vi "widget.vi"(8 "Error In":errorcluster, 10 "index":i32, 11 "QStackedWidget In":refnum<class "QStackedWidget.lvclass">) -> (0 "Error Out":errorcluster, 2 "Value":refnum<class "QWidget.lvclass">, 3 "QStackedWidget Out":refnum<class "QStackedWidget.lvclass">)   [LabVIEW 2014, in "QStackedWidget.lvclass"]
doc: "LabVIEW-specific documentation is not yet available. See <b>https://doc.qt.io/qt-5/qstackedwidget.html#widget</b>"
uses:
  QStackedWidget.lvclass
  QWidget/QWidget.lvclass
  LQ Core/LQIdentity/LQIdentity.lvclass/LQIdentity.ctl
  LQ Core/LQ Core.lvlib
  LQ Core/LQIdentity/LQIdentity.lvclass
  LQ Core/LQCoreEngine/LQCoreEngine.lvclass
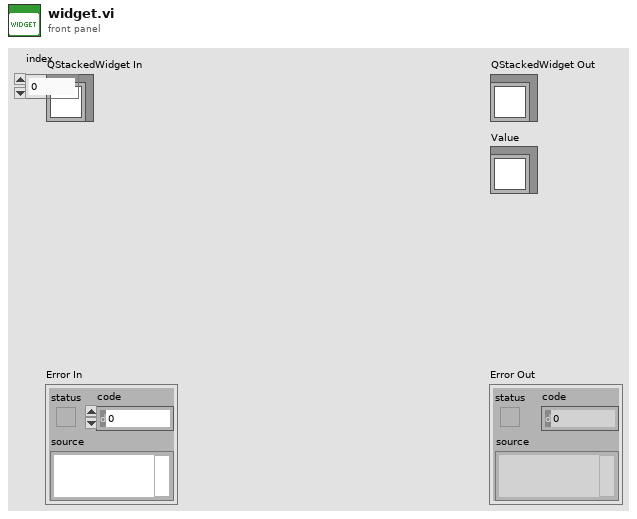
[diagram p1: front panel]
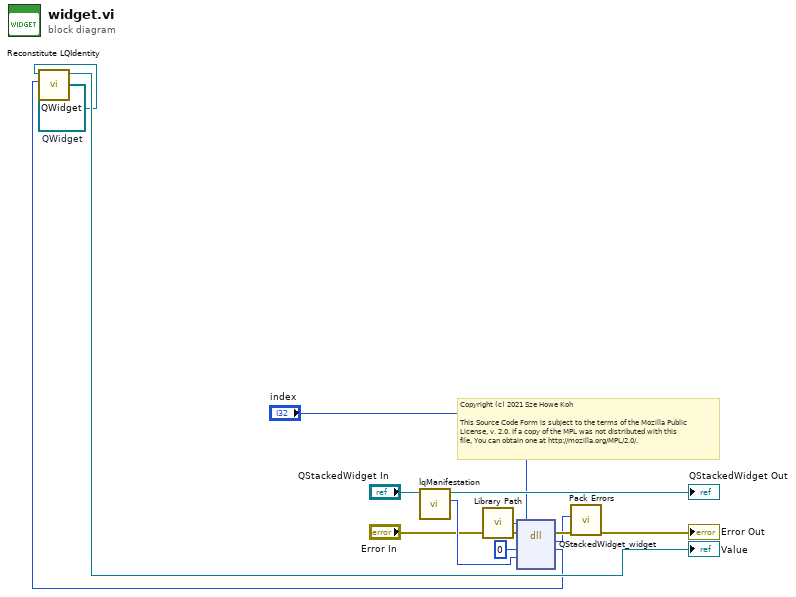
[diagram p0: block diagram]
diagram:
  w2 = refnum<class "QWidget.lvclass"> refnum  # QWidget
  # "Copyright (c) 2021 Sze Howe Koh\n\nThis Source Code Form is subject to the terms of the Mozilla Public\nLicense, v. 2.0. If a copy of the MPL was not distributed with this\nfile, You can obtain one at http://mozilla.org/MPL/2.0/."
  n1 = call "lqManifestation.vi"("LQIdentity in"="QStackedWidget In") -> ("Manifestation"=w9:u64, "LQIdentity out"=→"QStackedWidget Out":refnum<class "QStackedWidget.lvclass">)  [unwired: 9 in]
  n2 = call "Library Path.vi"() -> ("Library Path"=w10:path)
  n3 = dll-call lib="?" fn="QStackedWidget_widget"(path in=w10, error in="Error In", "_retVal"=u64 0 ("retVal"), "_instance"=w9, "index"="index") -> (error out=w7:errorcluster, w5:i32, "_retVal"=w3:u64)  [unwired: 3 in, 1 out]
  n4 = call "Reconstitute LQIdentity.vi"("Manifestation"=w3, "LQIdentity Prototype"=w2) -> ("Reconstituted LQIdentity"=→"Value":refnum<class "QWidget.lvclass">)  [unwired: 8 in, 1 out]
  n5 = call "Pack Errors.vi"("Error In"=w7, "Error Code"=w5) -> ("Error Out"=→"Error Out":errorcluster)  [unwired: 9 in]
